vi "ConvertChannelQueryResponseToEnable.vi"(8 "error in (no error)":errorcluster, 11 "TektronixDPO_PhysicalDevice.lvclass":refnum<class "TektronixDPO_PhysicalDevice.lvclass">) -> (0 "error out":errorcluster, 3 "TektronixDPO_PhysicalDevice.lvclassOut":refnum<class "TektronixDPO_PhysicalDevice.lvclass">)   [LabVIEW 2013, in "TektronixDPO_PhysicalDevice.lvclass"]
doc: "Read from the phsyical device the offset relative to the specified channel"
uses:
  TektronixDPO_PhysicalDevice.lvclass
  TektronixDPO_PhysicalDevice.lvclass/TektronixDPO_PhysicalDevice.ctl
panel:
  out "subarray":string[](array[string])
  # "Probe Gain"
  # "Bandwidth"
  # "Coupling"
  # "Offset"
  # "V/Division"
  # "Impedance"
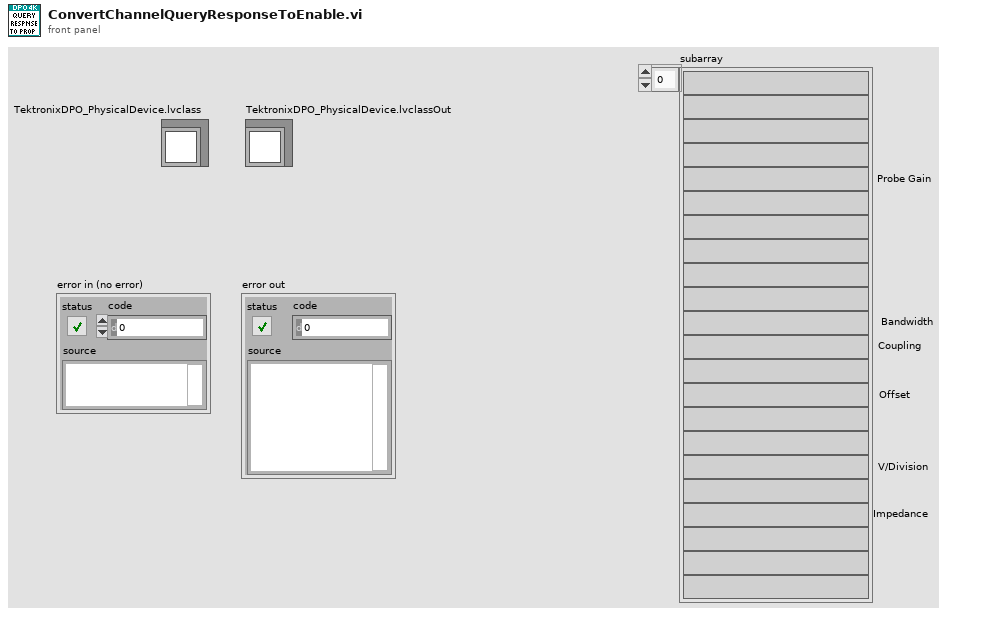
[diagram p1: front panel]
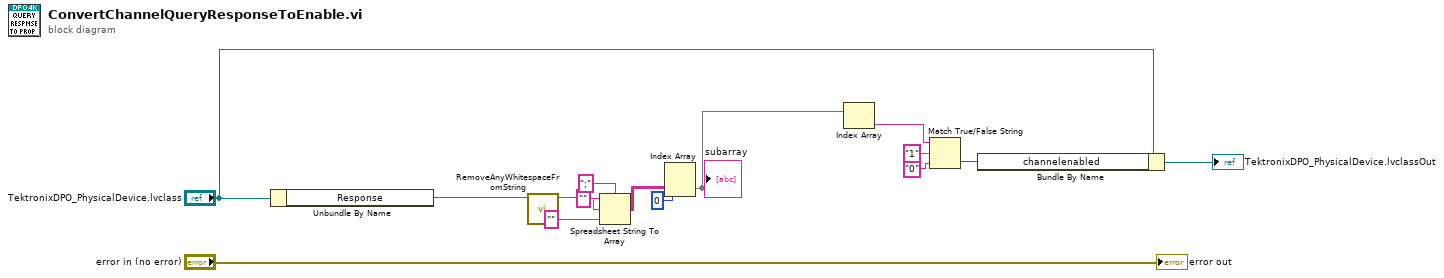
[diagram p0: block diagram]
diagram:
  n1 = Unbundle By Name("TektronixDPO_PhysicalDevice.lvclass") -> ("Response"=w6:string)
  n2 = call "RemoveAnyWhitespaceFromString.vi"("String in"=w6) -> ("String out"=w10:string)  [unwired: 10 in]
  n3 = Spreadsheet String To Array(delimiter (Tab)=";", format string="", spreadsheet string=w10, array type (2D Dbl)="") -> (array=w9:string[][])
  n4 = Index Array(array=w9, index (row)=0) -> (element=w7:string[])  [unwired: 1 in]
  "subarray" <- w7
  n5 = Index Array(array=w7) -> (element=w5:string)  [unwired: 1 in]
  n6 = Match True/False String(2:"0" ("false string"), 3:"1" ("true string"), 4:w5) -> (0:w2:bool)  [unwired: 1 out]
  n7 = Bundle By Name(cluster="TektronixDPO_PhysicalDevice.lvclass", "channelenabled"=w2) -> (→"TektronixDPO_PhysicalDevice.lvclassOut":refnum<class "TektronixDPO_PhysicalDevice.lvclass">)
  "error out" <- "error in (no error)"
